vi "getSamplingFsMode.vi"(8 "error in (no error)":errorcluster, 11 "Instrument.Lockin in":refnum<class "Instrument.Lockin.lvclass">) -> (0 "error out":errorcluster, 2 "Fs Mode":T1, 3 "Instrument.Lockin out":refnum<class "Instrument.Lockin.lvclass">)   [LabVIEW 2019, in "Instrument.Lockin.lvlib" / "Instrument.Lockin.lvclass"]
doc: "Returns the Sampling Fs Mode {Manual, Auto Fs, Max Fs} \n\nIf address=\"\", this API reads from localhost\nIf address is remote lockin, you need to add this computer to allowed whitelist on the lockin computer you are trying to access."
uses:
  Instrument.Lockin.lvclass
  <userlib>/LevyLab/Instrument Framework/Instrument Types/Lockin/Typedefs/LockinAPI.Sampling.FsMode--enum.ctl
  Typedefs/API/Lockin.Commands--Enum.ctl
  d8ce31b4-34f0-4bf6-9e65-fd5f51fc0a16.vi
  d8ce31b4-34f0-4bf6-9e65-fd5f51fc0a16.vi/83bdf9c3-7128-44d8-b601-7d848aa4e282.vi
  d8ce31b4-34f0-4bf6-9e65-fd5f51fc0a16.vi/838f9d0f-e6b5-4f3d-a03d-11fe12ead1f2.vi
  <vilib>/Utility/Data Type/Get Type Information.vi
  <vilib>/JDP Science/JSONtext/JSON text to Variant.vi
  <vilib>/JDP Science/JSONtext/LVClass Serializer/JSONtext LVClass Serializer.lvclass
  <userlib>/LevyLab/Instrument Framework/Instrument Types/Lockin/Instrument.LockinAPI.lvclass
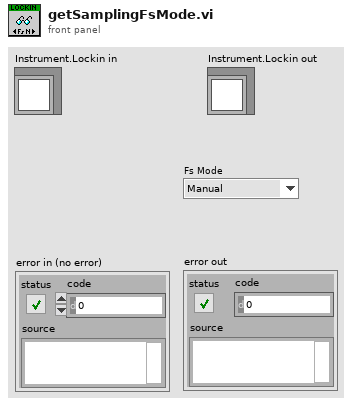
[diagram p1: front panel]
types:
  T1 = typedef "Instrument.LockinAPI.lvclass/LockinAPI.Sampling.FsMode--enum.ctl" = enum16{"Manual", "Auto Fs", "Max Fs"}
  T2 = typedef "Instrument.Lockin.lvlib/Instrument.Lockin.lvclass/Lockin.Commands--Enum.ctl" = enum16{"setAO", "setAO_Amplitude", "setAO_DC", "setAO_Frequency", "setAO_Phase", "setAO_Function", "setREF", "setREF_Frequency", "setREF_Phase", "setREF_TC", "setREF_Roll-Off", "setDAQ", "setSampling", "setState", "getState", "getAO", "getAI", "getResults", "getSampling", "getAOconfig", "getREFconfig", "setInputGain", "setOutputGain", "getInputGain", "getOutputGain", "setSamplingFsMode", "getSamplingFsMode", "setSweep", "setSweep_Time", "setSweep_Table", "getStatus", "getSweepResults", "getSweepWaveforms", "setLogMode"}
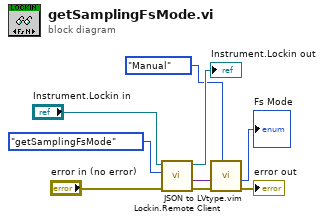
[diagram p0: block diagram]
diagram:
  n1 = call "Lockin.Remote Client.vi"("error in (no error)"="error in (no error)", "Command"=Lockin.Commands--Enum."getSamplingFsMode" ("Enum"), "Instrument.Lockin in"="Instrument.Lockin in") -> ("error out"=w5:errorcluster, "Data out"=w6:variant, "Instrument.Lockin out"=→"Instrument.Lockin out":refnum<class "Instrument.Lockin.lvclass">)  [unwired: 6 in]
  n2 = call "JSON to LVtype.vim"("type"=LockinAPI.Sampling.FsMode--enum."Manual" ("Fs Mode"), "error in (no error)"=w5, "JSON Data in"=w6) -> ("error out"=→"error out":errorcluster, "Data out"=→"Fs Mode":T1)  [unwired: 7 in]
